vi "Load NIPKG List from JSON File.vi"(8 "error in (no error)":errorcluster, 11 "file (use dialog)":path) -> (0 "error out":errorcluster, 3 "NIPKG List out":T1[](array[typedef]))   [LabVIEW 2017, in "NIPKG SBOM Support.lvlib"]
uses:
  NIPKG SBOM Support.lvlib
  <vilib>/National Instruments/NIPM API (Beta)/_support/package attributes.ctl
  d116f5af-0b28-470c-af4b-b547cd675569.vi
  <vilib>/JDP Science/JSONtext/JSON text to Variant.vi
  <vilib>/National Instruments/NIPM API (Beta)/NIPM_API.lvlib
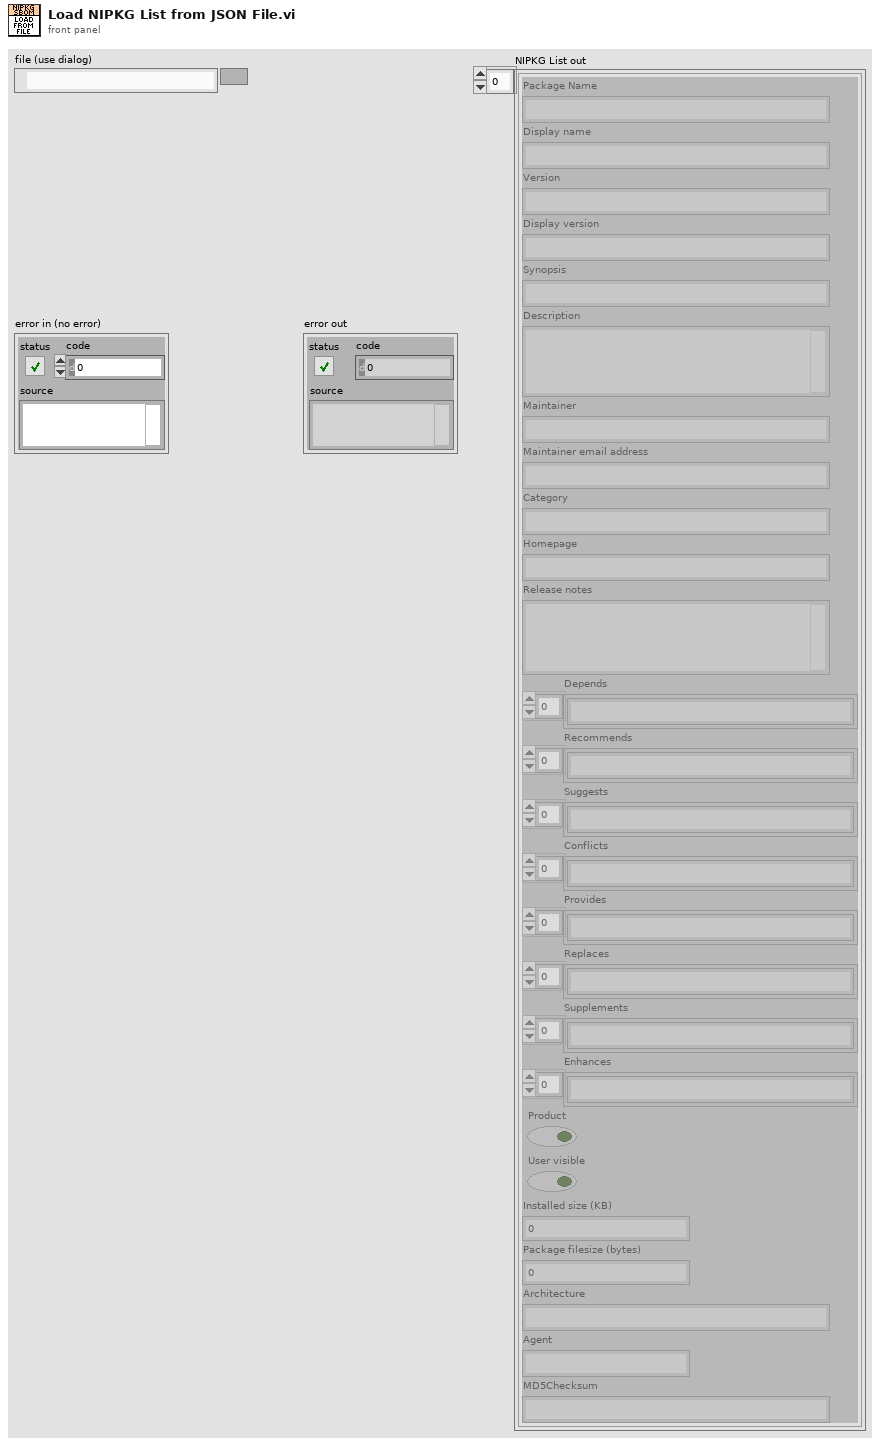
[diagram p1: front panel]
types:
  T1 = typedef "NIPM_API.lvlib/package attributes.ctl" = cluster{"Package Name":string, "Display name":string, "Version":string, "Display version":string, "Synopsis":string, "Description":string, "Maintainer":string, "Maintainer email address":string, "Category":string, "Homepage":string, "Release notes":string, "Depends":string[], "Recommends":string[], "Suggests":string[], "Conflicts":string[], "Provides":string[], "Replaces":string[], "Supplements":string[], "Enhances":string[], "Product":bool, "User visible":bool, "Installed size (KB)":u64, "Package filesize (bytes)":u64, "Architecture":string, "Agent":string, "MD5Checksum":string}
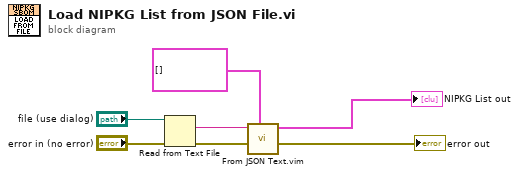
[diagram p0: block diagram]
diagram:
  n1 = Read from Text File(file (use dialog)="file (use dialog)", error in="error in (no error)") -> (text=w4:string, error out=w5:errorcluster)  [unwired: 2 in, 2 out]
  n2 = call "From JSON Text.vim"("Data Type and Default Value"=T1[] [] ("nipkg packages"), "error in (no error)"=w5, "JSON"=w4) -> ("error out"=→"error out":errorcluster, "Data out"=→"NIPKG List out":T1[])  [unwired: 7 in]
